vi "QMH_Enqueue_array.vi"(4 "Priority? (F)":bool, 6 "Queue_Ref":T1, 8 "error in (no error)":errorcluster, 10 "Payload":variant[](array[variant]), 11 "Message":string[](array[string])) -> (0 "error out":errorcluster)   [LabVIEW 2021, in "Framework_lib.lvlib"]
doc: "Enqueue element into the selected Queue"
uses:
  Framework_lib.lvlib
  QMH_references_enum.ctl
  framework_Qmessage.ctl
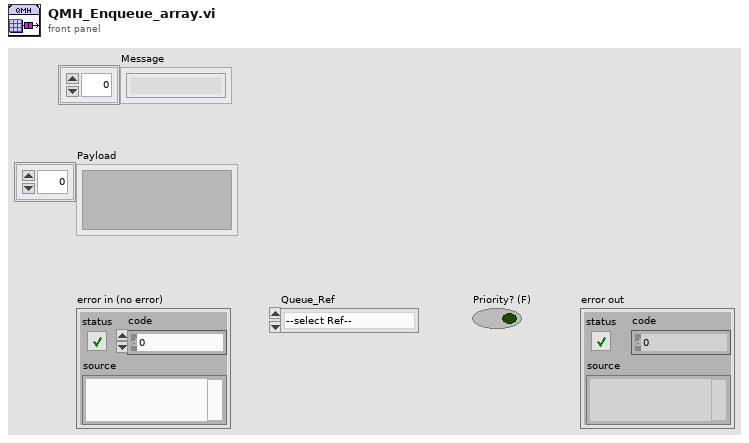
[diagram p1: front panel]
types:
  T1 = typedef "Framework_lib.lvlib/QMH_references_enum.ctl" = enum16{"--select Ref--", "Consumer_SUT", "Consumer_Annot", "Compute_Results"}
  T2 = typedef "Framework_lib.lvlib/framework_Qmessage.ctl" = cluster{"Message":string, "Payload":variant}
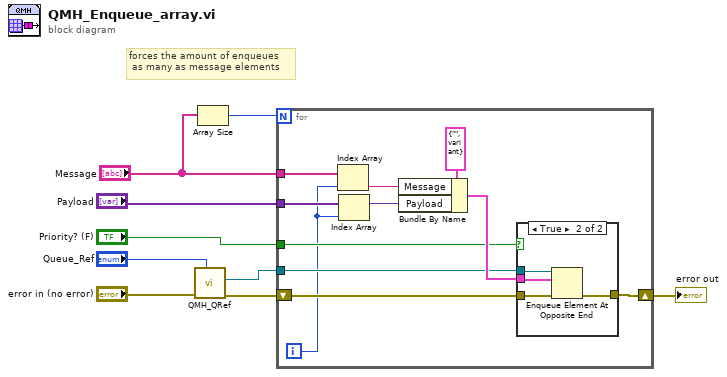
[diagram p0: block diagram]
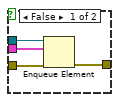
[diagram p2: hidden frame]
diagram:
  # "forces the amount of enqueues\n as many as message elements"
  n1 = call "QMH_QRef.vi"("Enum"="Queue_Ref", "error in (no error)"="error in (no error)") -> ("error out"=w7:errorcluster, "Queue_ref"=w5:refnum<queue>)  [unwired: 7 in, 1 out]
  n2 = Array Size(array="Message") -> (size(s)=w1:i32)
  n3 = for {
    N: w1 -> [_]
    tunnel: "Payload" -> [w16]
    tunnel: w5 -> [w15]
    tunnel: "Priority? (F)" -> [w14]
    shift-right: [w20] -> w9
    shift-left: w7 -> [w17]
    tunnel: "Message" -> [w13]
    i -> [w10]
    n4 = Index Array(array=w13, index=w10) -> (element=w11:string)
    n5 = Index Array(array=w16, index=w10) -> (element=w12:variant)
    n6 = Bundle By Name(cluster=T2 {"Message"="", "Payload"=variant} ("element"), "Message"=w11, "Payload"=w12) -> (w18:T2)
    n7 = case shown="True" w14 {
      tunnel: [w24 w27] -> w20
      tunnel: w18 -> [w23 w26]
      tunnel: w17 -> [w22 w28]
      tunnel: w15 -> [w21 w25]
      frame False {
        n8 = Enqueue Element(queue=w21, element=w23, error in (no error)=w22) -> (error out=w24:errorcluster)  [unwired: 1 in, 2 out]
      }
      frame True {
        n9 = Enqueue Element At Opposite End(queue=w25, element=w26, error in (no error)=w28) -> (error out=w27:errorcluster)  [unwired: 1 in, 2 out]
      }
    }
  }
  "error out" <- w9
